vi "Create Parameters.vi"(8 "error in (no error)":errorcluster, 11 "Controls References Hash":variant) -> (0 "error out":errorcluster, 3 "Parameters Map":variant)   [LabVIEW 2013, in "File IO.lvlib"]
uses:
  File IO.lvlib
  Parameter/Sensor Parameter/Sensor Parameter.lvclass
  Parameter/Abstract Sensor Parameter/Abstract Sensor Parameter.lvclass
  Parameter/Abstract Sensor Parameter/Abstract Sensor Parameter.lvclass/Abstract Sensor Parameter.ctl
  Control Reference/Control Reference.lvlib
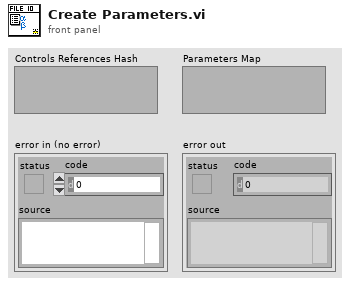
[diagram p1: front panel]
types:
  T1 = enum8{"Enabled", "Disabled", "Disabled and Grayed Out"}
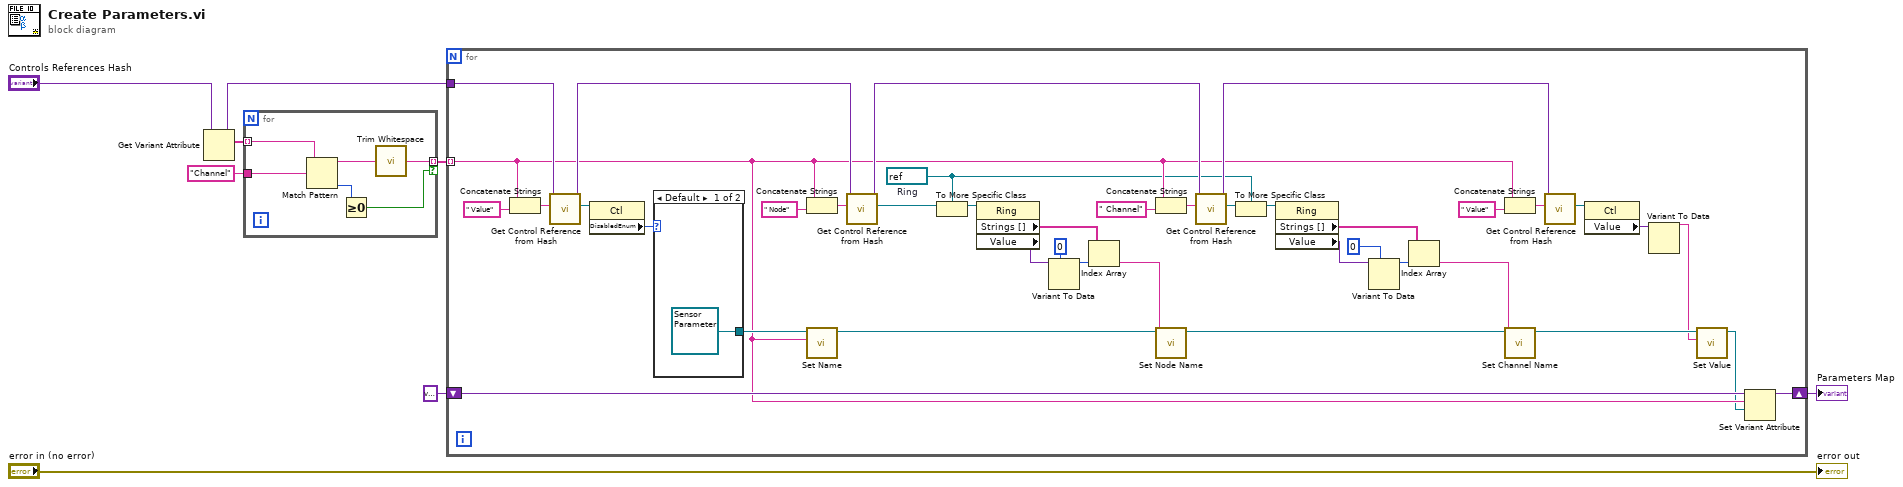
[diagram p0: block diagram]
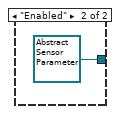
[diagram p2: hidden frame]
diagram:
  n1 = Get Variant Attribute(Variant="Controls References Hash") -> (duplicate Variant=w4:variant, names=w8:string[])  [unwired: 3 in, 2 out]
  n2 = for {
    tunnel: w8 -> [w12] mode=indexing
    tunnel: "Channel" -> [w13]
    tunnel: [w10] -> w6 mode=indexing if=w9
    n3 = Match Pattern(string=w12, regular expression=w13) -> (before substring=w11:string, offset past match=w14:i32)  [unwired: 1 in, 2 out]
    n4 = Greater Or Equal To 0?(x=w14) -> (x >= 0?=w9:bool)
    n5 = call <vilib>:"Trim Whitespace.vi"("string"=w11) -> ("trimmed string"=w10:string)  [unwired: 1 in]
  }
  n6 = for {
    tunnel: w4 -> [w50]
    tunnel: w6 -> [w29] mode=indexing
    shift-right: [w30] -> w1
    shift-left: variant ("variant") -> [w31]
    w26 = refnum<vi> refnum  # Ring
    n7 = Concatenate Strings(w29, " Value" ("string")) -> (w52:string)
    n8 = call "Get Control Reference from Hash.vi"("control label"=w52, "controls references hash"=w50) -> ("control reference"=w54:refnum<vi>, "duplicated controls references hash"=w39:variant)  [unwired: 6 in, 2 out]
    n9 = property class="Ctl"(reference=w54) -> ("DisabledEnum"=w51:T1)  [unwired: 1 in, 2 out]
    n10 = case shown="Default" w51 {
      tunnel: [refnum<class "Sensor Parameter.lvclass"> refnum ("Parameter.lvlib:Sensor Parameter.lvclass") refnum<class "Abstract Sensor Parameter.lvclass"> refnum ("Parameter.lvlib:Abstract Sensor Parameter.lvclass")] -> w49
      frame Default {
      }
      frame "Enabled" {
      }
    }
    n11 = Concatenate Strings(w29, " Node" ("string")) -> (w48:string)
    n12 = call "Set Name.vi"("Name"=w29, "Parameter in"=w49) -> ("Parameter out"=w45:refnum<class "Abstract Sensor Parameter.lvclass">)  [unwired: 8 in, 1 out]
    n13 = call "Get Control Reference from Hash.vi"("control label"=w48, "controls references hash"=w39) -> ("control reference"=w46:refnum<vi>, "duplicated controls references hash"=w34:variant)  [unwired: 6 in, 2 out]
    n14 = To More Specific Class(target class=w26, reference=w46) -> (specific class reference=w27:refnum<vi>)  [unwired: 1 in, 1 out]
    n15 = property class="Ring"(reference=w27) -> ("Strings []"=w24:string[], "Value"=w25:variant)  [unwired: 1 in, 2 out]
    n16 = Variant To Data(type=0, Variant=w25) -> (data=w22:i32)  [unwired: 1 in, 1 out]
    n17 = Index Array(array=w24, index=w22) -> (element=w21:string)
    n18 = Concatenate Strings(w29, " Channel" ("string")) -> (w40:string)
    n19 = call "Set Node Name.vi"("Node Name"=w21, "Parameter in"=w45) -> ("Parameter out"=w44:refnum<class "Abstract Sensor Parameter.lvclass">)  [unwired: 8 in, 1 out]
    n20 = call "Get Control Reference from Hash.vi"("control label"=w40, "controls references hash"=w34) -> ("control reference"=w42:refnum<vi>, "duplicated controls references hash"=w33:variant)  [unwired: 6 in, 2 out]
    n21 = To More Specific Class(target class=w26, reference=w42) -> (specific class reference=w16:refnum<vi>)  [unwired: 1 in, 1 out]
    n22 = property class="Ring"(reference=w16) -> ("Strings []"=w19:string[], "Value"=w20:variant)  [unwired: 1 in, 2 out]
    n23 = Variant To Data(type=0, Variant=w20) -> (data=w17:i32)  [unwired: 1 in, 1 out]
    n24 = Index Array(array=w19, index=w17) -> (element=w15:string)
    n25 = Concatenate Strings(w29, " Value" ("string")) -> (w38:string)
    n26 = call "Set Channel Name.vi"("Channel Name"=w15, "Parameter in"=w44) -> ("Parameter out"=w43:refnum<class "Abstract Sensor Parameter.lvclass">)  [unwired: 8 in, 1 out]
    n27 = call "Get Control Reference from Hash.vi"("control label"=w38, "controls references hash"=w33) -> ("control reference"=w36:refnum<vi>)  [unwired: 6 in, 3 out]
    n28 = property class="Ctl"(reference=w36) -> ("Value"=w35:variant)  [unwired: 1 in, 2 out]
    n29 = Variant To Data(Variant=w35) -> (data=w32:string)  [unwired: 2 in, 1 out]
    n30 = call "Set Value.vi"("Value"=w32, "Parameter in"=w43) -> ("Parameter out"=w28:refnum<class "Abstract Sensor Parameter.lvclass">)  [unwired: 8 in, 1 out]
    n31 = Set Variant Attribute(Variant=w31, name=w29, value=w28) -> (Variant out=w30:variant)  [unwired: 1 in, 2 out]
  }
  "Parameters Map" <- w1
  "error out" <- "error in (no error)"
